vi "Move Steps.vi"(8 "error in (no error)":errorcluster, 9 "Number Of Steps":T1, 10 "Model in":refnum<class "Model.lvclass">, 11 "State in":refnum<class "State.lvclass">) -> (0 "error out":errorcluster, 2 "Model out":refnum<class "Model.lvclass">, 3 "State out":refnum<class "State.lvclass">)   [LabVIEW 2016, in "State.lvclass"]
uses:
  State.lvclass
  Model/Model/Model.lvclass
  Typedefs/Number Of Steps.ctl
  Typedefs/HPMT_Typedefs.lvlib
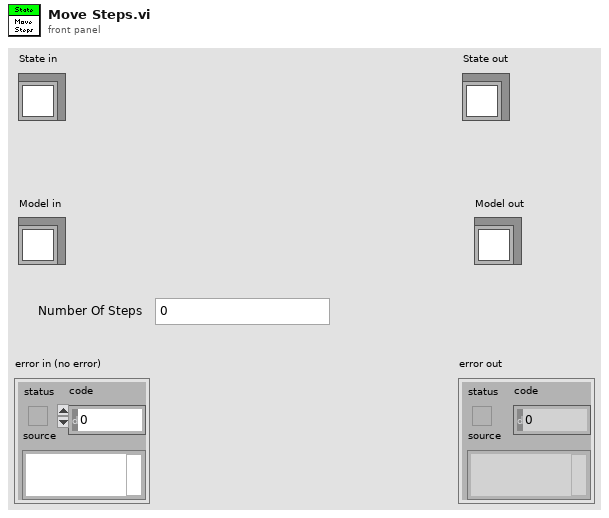
[diagram p1: front panel]
types:
  T1 = typedef "HPMT_Typedefs.lvlib/Number Of Steps.ctl" = i32
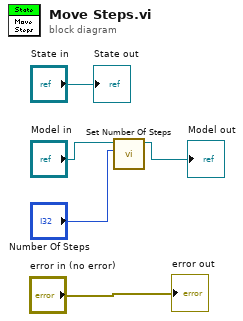
[diagram p0: block diagram]
diagram:
  n1 = call "Set Number Of Steps.vi"("Number Of Steps"="Number Of Steps", "Model in"="Model in") -> ("Model out"=→"Model out":refnum<class "Model.lvclass">)  [unwired: 9 in]
  "error out" <- "error in (no error)"
  "State out" <- "State in"
